vi "Remove Specific Char from Signal Name.vi"(0 "reference in":refnum<class "GSwFormDSP.lvclass">, 5 "error in (no error)":errorcluster, 7 "Characters to remove":string[](array[string]), 9 "Replace with":string=" ") -> (14 "reference out":refnum<class "GSwFormDSP.lvclass">, 19 "error out":errorcluster)   [LabVIEW 2020, in "GSwFormDSP.lvclass"]
uses:
  GSwFormDSP.lvclass
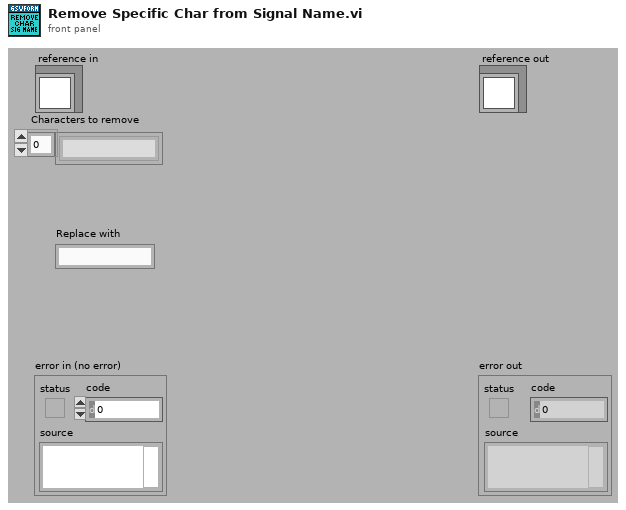
[diagram p1: front panel]
types:
  T1 = typedef "GSwFormDSP.lvclass/ObjectAttributesRef.ctl" = refnum<data-value>
  T2 = typedef "GSwFormDSP.lvclass/ObjectAttributes.ctl" = cluster{"Wform Ref":refnum<data-value>, "Nb Signals":i32, "Spectral Function Parameters":T3, "FFT":waveform(cdb)[], "Nb FFT":i32, "Nb Averages":i32[], "Reference Indexes":i32[], "Response Indexes":i32[], "Coherence":waveform(dbl)[], "TDF Parameters":T5, "DAQ":cluster{"Duration (sec)":dbl, "Buffer Size (Samples)":i32, "Offset (Samples)":i32}, "Filter Impulse Response (TDF)":waveform(dbl), "Sound Playback":T6}
  T3 = typedef "GSwFormDSP.lvclass/Spectral Parameters.ctl" = cluster{"Frequency resolution (Hz)":dbl, "Overlap":dbl, "Window":T4}
  T4 = typedef "NI_AALPro.lvlib/windowTd.ctl" = u32
  T5 = typedef "GSwFormDSP.lvclass/TDF Parameters.ctl" = cluster{"Filter":enum32{"Lowpass", "Highpass", "Bandpass", "Bandstop"}, "Type:":enum16{"Butterworth", "Chebyshev", "Inv Chebyshev", "Elliptic", "Bessel"}, "LP cutoff freq":dbl, "HP cutoff freq":dbl, "Order":i32, "passband ripple (dB)":dbl, "stopband attenuation (dB)":dbl, "Phaseless Filter":bool, "Include Fade IN and OUT":bool}
  T6 = typedef "GSwFormDSP.lvclass/Sound Playback.ctl" = cluster{"Timer start (ms)":u32, "task ID":T7, "Cursor Init Location (s)":dbl, "SC Volume":dbl}
  T7 = typedef "Sound Output Task ID.ctl" = u32
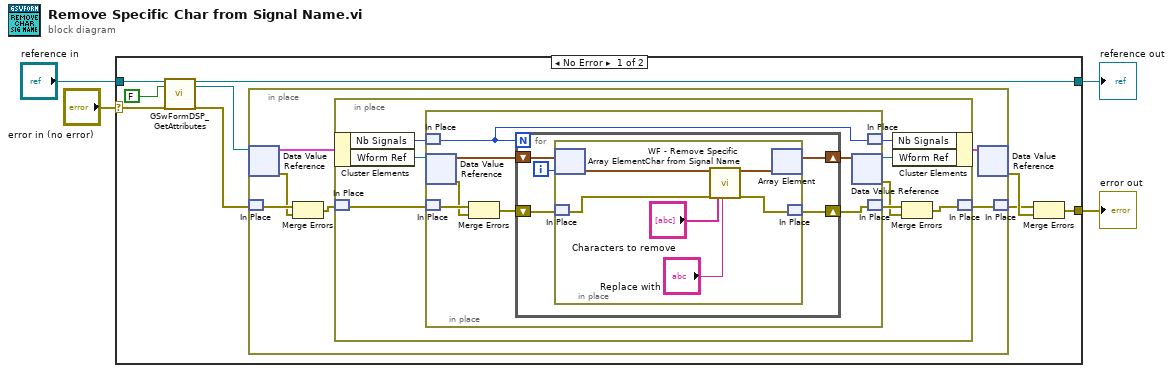
[diagram p0: block diagram]
diagram:
  n1 = case shown="No Error" "error in (no error)" {
    selector: "error in (no error)" -> [w9 w47]
    tunnel: [w13 w47] -> w4
    tunnel: [w8 w46] -> w2
    tunnel: "reference in" -> [w11 w46]
    frame No Error {
      n2 = call "GSwFormDSP_GetAttributes.vi"("reference in"=w11, "return data? (T)"=FALSE, "error in (no error)"=w9) -> ("reference out"=w8:refnum<class "GSwFormDSP.lvclass">, "attributes ref"=w7:T1, "error out"=w6:errorcluster)  [unwired: 13 in, 1 out]
      n3 = in-place {
        n4 = in-place-dvr #1(w7) -> (w18:T2, w16:errorcluster)
        n5 = in-place-match #2(w6) -> (w17:errorcluster)
        n6 = Merge Errors(w17, w16) -> (w15:errorcluster)
        n7 = in-place {
          n8 = in-place-cluster #3(w18) -> ("Nb Signals"=w21:i32, "Wform Ref"=w27:refnum<data-value>)
          n9 = in-place-match #4(w15) -> (w25:errorcluster)
          n10 = in-place {
            n11 = in-place-match #5(w21) -> (w28:i32)
            n12 = in-place-dvr #6(w27) -> (w34:waveform(dbl)[], w32:errorcluster)
            n13 = in-place-match #7(w25) -> (w33:errorcluster)
            n14 = Merge Errors(w33, w32) -> (w29:errorcluster)
            n15 = for {
              N: w28 -> [_]
              shift-right: [w38] -> w31
              shift-left: w34 -> [w39]
              shift-right: [w35] -> w30
              shift-left: w29 -> [w36]
              i -> [w37]
              n16 = in-place {
                n17 = in-place-array #8(w39, w37) -> (w45:waveform(dbl))
                n18 = in-place-match #9(w36) -> (w43:errorcluster)
                n19 = call "WF - Remove Specific Char from Signal Name.vi"("wForm IN"=w45, "error in (no error)"=w43, "Characters to remove"="Characters to remove", "Replace with"="Replace with") -> ("wForm OUT"=w44:waveform(dbl), "error out"=w42:errorcluster)  [unwired: 14 in]
                n20 = in-place-array #8(w44) -> (w38:waveform(dbl)[])  [unwired: 1 out]
                n21 = in-place-match #9(w42) -> (w35:errorcluster)
              }
            }
            n22 = in-place-dvr #6(w31) -> (w26:refnum<data-value>, w23:errorcluster)
            n23 = in-place-match #5(w28) -> (w20:i32)
            n24 = in-place-match #7(w30) -> (w24:errorcluster)
          }
          n25 = in-place-cluster #3("Nb Signals"=w20, "Wform Ref"=w26) -> (w19:T2)
          n26 = Merge Errors(w24, w23) -> (w22:errorcluster)
          n27 = in-place-match #4(w22) -> (w14:errorcluster)
        }
        n28 = in-place-dvr #1(w19) -> (w12:errorcluster)  [unwired: 1 out]
        n29 = in-place-match #2(w14) -> (w5:errorcluster)
      }
      n30 = Merge Errors(w5, w12) -> (w13:errorcluster)
    }
    frame Error {
    }
  }
  "error out" <- w4
  "reference out" <- w2
